vi "BLM Control Act.vi"(0 "command text in":string[](array[string])) -> ()   [LabVIEW 2019]
uses:
  VI Server Control N1/VI Server Control.ctl
panel:
  in  "VI Server Control":T1={"VI name"="", "Control"=[], "Value"=[], "Boolean?"=[], "Control to End"="", "Condition"=enum."within xxx% of target value", "xxx%"=0.0, "Target Value"=0.0, "Timeout (sec)"=120.0, "wait (sec)"=120.0, "check every (s)"=120.0, "Boolean indi"=FALSE} {"Boolean?" min=0.0 max=1.0 step=1.0 format="%#_1g"}
  # "0"
  # "1"
  # "2"
  # "3"
  # "4"
  # "5"
  # "6"
  # "7"
  # "8"
  # "9"
  # "Finish if"
  # "is"
  # "and also finish the whole thing if time elapses"
  # "or longer."
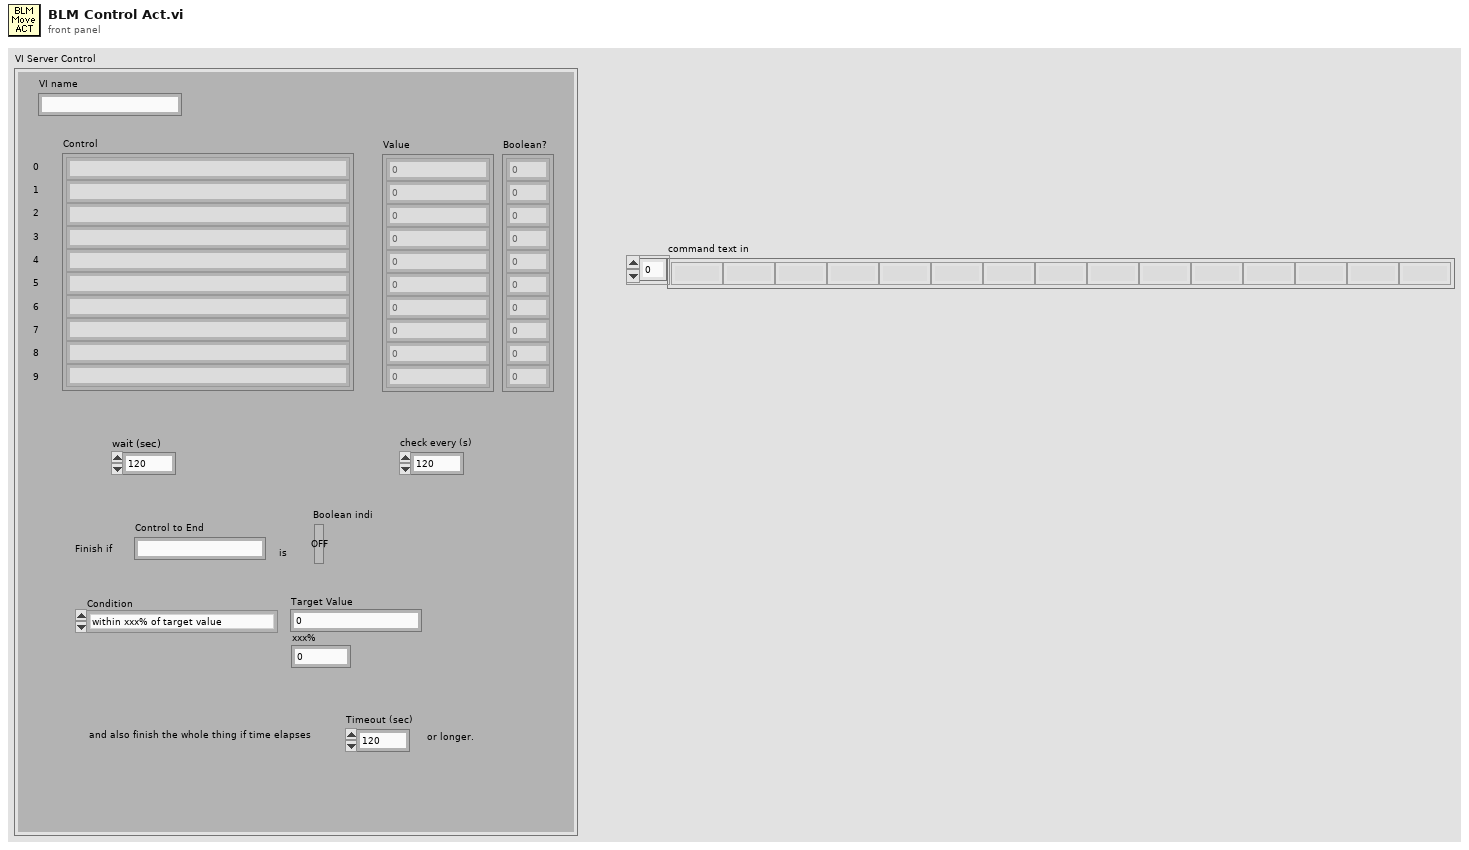
[diagram p1: front panel]
types:
  T1 = typedef "VI Server Control.ctl" = cluster{"VI name":string, "Control":string[], "Value":dbl[], "Boolean?":dbl[], "Control to End":string, "Condition":enum16{"within xxx% of target value", "<= target value", ">= target value", "= target value"}, "xxx%":dbl, "Target Value":dbl, "Timeout (sec)":dbl, "wait (sec)":dbl, "check every (s)":dbl, "Boolean indi":bool}
  T2 = typedef "Stepper Mover.ctl" = cluster{"extra wait":i32, "Stepper Value":dbl, "Top or Bottom":enum32{"Move to Top Position (deg)", "Move to Bottom Position (deg or in)"}}
  T3 = enum16{"within xxx% of target value", "<= target value", ">= target value", "= target value"}
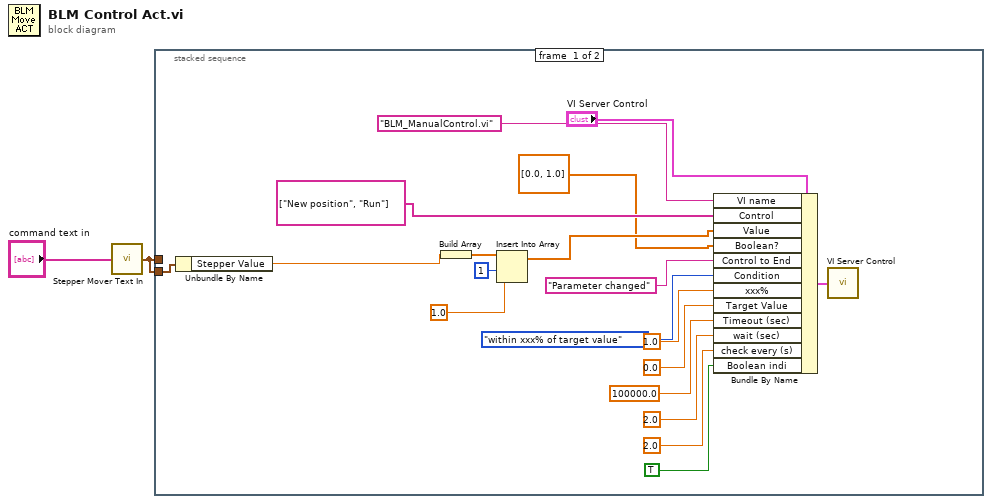
[diagram p0: block diagram]
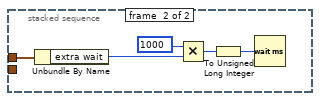
[diagram p2: hidden frame]
diagram:
  n1 = call "Stepper Mover Text In.vi"("command text in"="command text in") -> ("Stepper Mover"=w2:T2)
  n2 = stacked-sequence {
    tunnel: w2 -> [w21 _]
    tunnel: w2 -> [_ w23]
    frame #0 {
      n3 = Unbundle By Name(w21) -> ("Stepper Value"=w8:dbl)
      n4 = Build Array(w8) -> (w7:dbl[])
      n5 = Insert Into Array(array=w7, index=1, new element=1.0 ("new element/subarray")) -> (w4:dbl[])
      n6 = Bundle By Name(cluster="VI Server Control", "VI name"="BLM_ManualControl.vi", "Control"=string[] ["New position", "Run"], "Value"=w4, "Boolean?"=dbl[] [0.0, 1.0], "Control to End"="Parameter changed", "Condition"=T3."within xxx% of target value", "xxx%"=1.0, "Target Value"=0.0, "Timeout (sec)"=100000.0, "wait (sec)"=2.0, "check every (s)"=2.0, "Boolean indi"=TRUE) -> (w20:T1)
      n7 = call "VI Server Control.vi"("VI Server Control"=w20) -> ()
    }
    frame #1 {
      n8 = Unbundle By Name(w23) -> ("extra wait"=w22:i32)
      n9 = Multiply(x=1000 ("y"), y=w22) -> (x*y=w25:i32)
      n10 = To Unsigned Long Integer(number=w25) -> (unsigned 32bit integer=w24:u32)
      n11 = Wait (ms)(milliseconds to wait=w24) -> ()  [unwired: 1 out]
    }
  }
